vi "StraightCurveX.vi"(11 "9dots":dbl[][](array[numeric])) -> (3 "曲面调整":dbl)   [LabVIEW 2011]
uses:
  <vilib>/vision/NI_Vision_Development_Module.lvlib
  <vilib>/Analysis/NI_AALBase.lvlib
panel:
  out "添加的数组":dbl[](array[numeric])
  out "交织的数组":sgl[](array[numeric])
  out "Distances":sgl[](array[numeric]) format="%.4f"
  out "Distances 2":sgl[](array[numeric]) format="%.4f"
  out "Distances 3":sgl[](array[numeric]) format="%.4f"
  out "r":dbl
  out "detaY":dbl caption="均值" format="%0.2f"
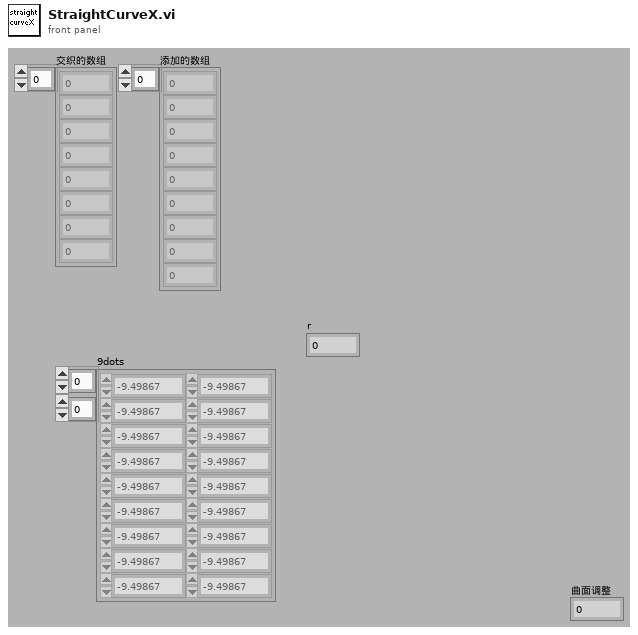
[diagram p1: front panel]
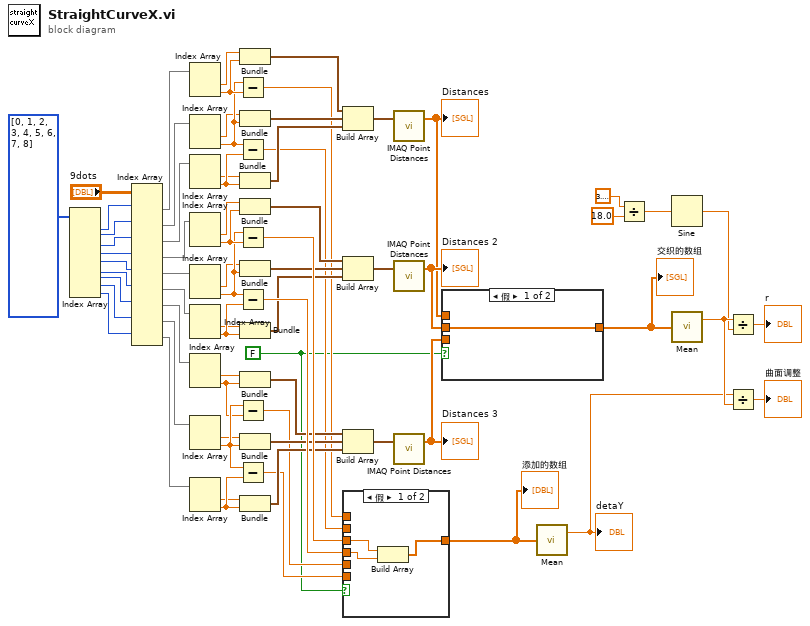
[diagram p0: block diagram]
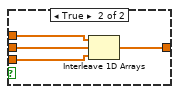
[diagram p2: hidden frame]
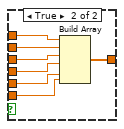
[diagram p3: hidden frame]
diagram:
  w1 = FALSE
  n1 = Index Array(array=i32[] [0, 1, 2, 3, 4, 5, 6, 7, 8] ("Distances 4")) -> (element #1=w15:i32, element #2=w14:i32, element #3=w13:i32, element #4=w12:i32, element #5=w11:i32, element #6=w10:i32, element #7=w9:i32, element #8=w8:i32, element #9=w7:i32)  [unwired: 9 in]
  n2 = Index Array(array="9dots", index (row) #1=w15, index (row) #2=w14, index (row) #3=w13, index (row) #4=w12, index (row) #5=w11, index (row) #6=w10, index (row) #7=w9, index (row) #8=w8, index (row) #9=w7) -> (element #1=w17:dbl[], element #2=w27:dbl[], element #3=w28:dbl[], element #4=w29:dbl[], element #5=w30:dbl[], element #6=w31:dbl[], element #7=w32:dbl[], element #8=w33:dbl[], element #9=w34:dbl[])  [unwired: 9 in]
  n3 = Index Array(array=w17) -> (element #1=w18:dbl, element #2=w56:dbl)  [unwired: 2 in]
  n4 = Index Array(array=w27) -> (element #1=w19:dbl, element #2=w55:dbl)  [unwired: 2 in]
  n5 = Index Array(array=w28) -> (element #1=w20:dbl, element #2=w57:dbl)  [unwired: 2 in]
  n6 = Index Array(array=w29) -> (element #1=w21:dbl, element #2=w59:dbl)  [unwired: 2 in]
  n7 = Index Array(array=w30) -> (element #1=w22:dbl, element #2=w58:dbl)  [unwired: 2 in]
  n8 = Index Array(array=w31) -> (element #1=w23:dbl, element #2=w60:dbl)  [unwired: 2 in]
  n9 = Index Array(array=w32) -> (element #1=w24:dbl, element #2=w61:dbl)  [unwired: 2 in]
  n10 = Index Array(array=w33) -> (element #1=w25:dbl, element #2=w65:dbl)  [unwired: 2 in]
  n11 = Index Array(array=w34) -> (element #1=w26:dbl, element #2=w62:dbl)  [unwired: 2 in]
  n12 = Subtract(x=w55, y=w56) -> (x-y=w5:dbl)
  n13 = Subtract(x=w55, y=w57) -> (x-y=w4:dbl)
  n14 = Subtract(x=w58, y=w59) -> (x-y=w63:dbl)
  n15 = Subtract(x=w58, y=w60) -> (x-y=w64:dbl)
  n16 = Subtract(x=w65, y=w61) -> (x-y=w3:dbl)
  n17 = Subtract(x=w65, y=w62) -> (x-y=w2:dbl)
  n18 = Bundle("Numeric"=w18, "Numeric"=w56) -> (w35:cluster{"Numeric":dbl, "Numeric":dbl})  [unwired: 1 out]
  n19 = Bundle("Numeric"=w19, "Numeric"=w55) -> (w36:cluster{"Numeric":dbl, "Numeric":dbl})  [unwired: 1 out]
  n20 = Bundle("Numeric"=w20, "Numeric"=w57) -> (w37:cluster{"Numeric":dbl, "Numeric":dbl})  [unwired: 1 out]
  n21 = Bundle("Numeric"=w21, "Numeric"=w59) -> (w38:cluster{"Numeric":dbl, "Numeric":dbl})  [unwired: 1 out]
  n22 = Bundle("Numeric"=w22, "Numeric"=w58) -> (w39:cluster{"Numeric":dbl, "Numeric":dbl})  [unwired: 1 out]
  n23 = Bundle("Numeric"=w23, "Numeric"=w60) -> (w40:cluster{"Numeric":dbl, "Numeric":dbl})  [unwired: 1 out]
  n24 = Bundle("Numeric"=w24, "Numeric"=w61) -> (w41:cluster{"Numeric":dbl, "Numeric":dbl})  [unwired: 1 out]
  n25 = Bundle("Numeric"=w25, "Numeric"=w65) -> (w42:cluster{"Numeric":dbl, "Numeric":dbl})  [unwired: 1 out]
  n26 = Bundle("Numeric"=w26, "Numeric"=w62) -> (w43:cluster{"Numeric":dbl, "Numeric":dbl})  [unwired: 1 out]
  n27 = Build Array(w35, w36, w37) -> (w44:cluster{"Numeric":dbl, "Numeric":dbl}[])
  n28 = Build Array(w38, w39, w40) -> (w45:cluster{"Numeric":dbl, "Numeric":dbl}[])
  n29 = Build Array(w41, w42, w43) -> (w46:cluster{"Numeric":dbl, "Numeric":dbl}[])
  n30 = case shown="假" w1 {
    tunnel: [w71 w80] -> w66
    tunnel: w64 -> [w72 w79]
    tunnel: w63 -> [w73 w78]
    tunnel: w5 -> [_ w77]
    tunnel: w4 -> [_ w76]
    tunnel: w3 -> [_ w75]
    tunnel: w2 -> [_ w74]
    frame False {
      n31 = Build Array(w73, w72) -> (w71:dbl[])
    }
    frame True {
      n32 = Build Array(w77, w76, w78, w79, w75, w74) -> (w80:dbl[])
    }
  }
  "添加的数组" <- w66
  n33 = call "IMAQ Point Distances"("Points"=w44) -> ("Distances"=w47:sgl[])  [unwired: 1 in, 4 out]
  "Distances" <- w47
  n34 = call "IMAQ Point Distances"("Points"=w45) -> ("Distances"=w48:sgl[])  [unwired: 1 in, 4 out]
  "Distances 2" <- w48
  n35 = call "IMAQ Point Distances"("Points"=w46) -> ("Distances"=w49:sgl[])  [unwired: 1 in, 4 out]
  "Distances 3" <- w49
  n36 = case shown="假" w1 {
    tunnel: [w81 w85] -> w50
    tunnel: w49 -> [_ w84]
    tunnel: w48 -> [w81 w83]
    tunnel: w47 -> [_ w82]
    frame False {
    }
    frame True {
      n37 = Interleave 1D Arrays(w82, w83, w84) -> (w85:sgl[])
    }
  }
  "交织的数组" <- w50
  n38 = call <vilib>:"Mean.vi"("X"=w66) -> ("mean"=w67:dbl)  [unwired: 1 out]
  "detaY" <- w67
  n39 = Divide(x=3.141592653589793, y=18.0) -> (x/y=w54:dbl)
  n40 = Sine(x=w54) -> (sin(x)=w51:dbl)
  n41 = call <vilib>:"Mean.vi"("X"=w50) -> ("mean"=w69:dbl)  [unwired: 1 out]
  n42 = Divide(x=w69, y=w51) -> (x/y=→"r":dbl)
  n43 = Divide(x=w67, y=w69) -> (x/y=→"曲面调整":dbl)
